vi "ExEMCircBufKinetics.vi"() -> ()   [LabVIEW 2010]
uses:
  CamHandle.vi
panel:
  out "Current clock index":u32
  out "current clock value":dbl format="%.2f"
  out "Min Clock index":u32
  out "Max Clock index":u32
  in  "Enum":T1(ring)
  in  "Vertical Clock":u32=2 min=1 max=16 step=1
  in  "Window Size":u32=50 min=1 step=1
  in  "av gain":dbl format="%.2f"
  in  "Invert Logic output":bool
  in  "Logic Output":i32
  in  "Fan":i32=1
  in  "ADC Gain":u32
  out "ADC Speed (Khz)":u32
  in  "Fast ADC":bool
  in  "Temperature":dbl=-70.0 format="%.2f"
  in  "Exposure":dbl min=0.0 step=0.001 format="%.3f"
  in  "stop":bool
  in  "Store":bool
  out "error out":errorcluster
  in  "error in (no error)":errorcluster
  # "ExEMCircBufKinetics:\nThis example allows a full image\nto be programmed up. It then runs\nin sync (focus) and kinetics mode displaying the full image made up\nof kinetic window exposures.\nNote: this example requires the \ncamera support circular buffers.\nThis example also shows how to \nsetup the cascade to run in over-\nlapped mode and how to set the\non-chip multiplication gain and how\nto set the readout port."
  # "Warning: you must open and run once the VI ExOpenGlobalCam.vi.\nYou only need to run it once then you can run this Example VI as many\ntimes as you want."
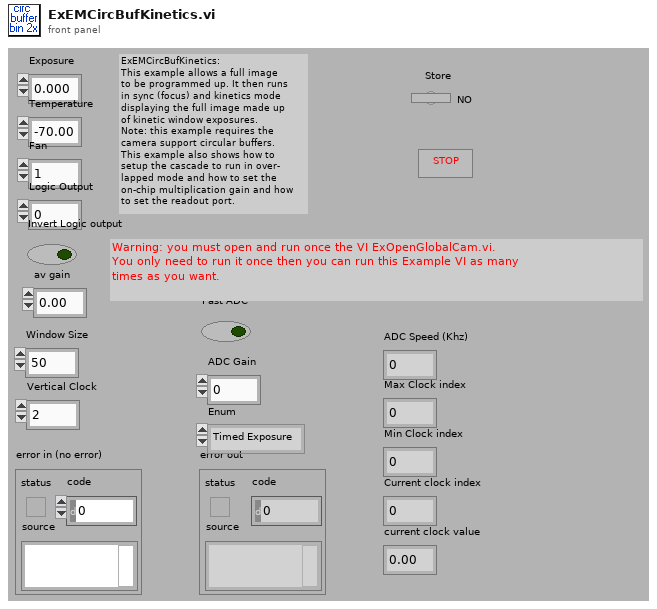
[diagram p1: front panel]
types:
  T1 = enum32{"Timed Exposure", "Trigger Once", "Trigger Multiple", "Trigger Bulb"}
  T2 = cluster{"Camera Handle":u32, "File Handle":u32, "Display Handle":u32, "Image Handle":u32}
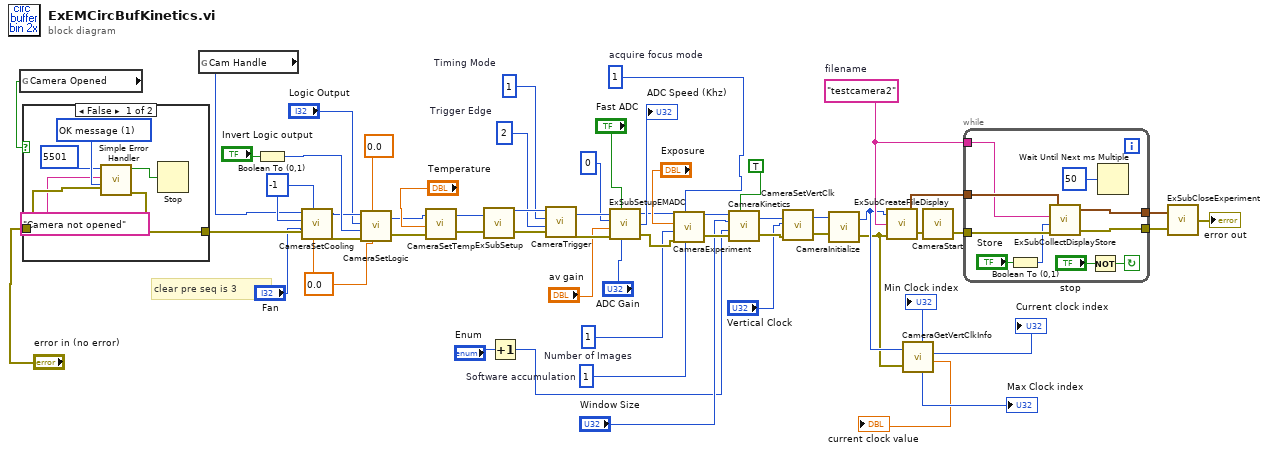
[diagram p0: block diagram]
diagram:
  w30 = 0.0
  w31 = -1
  w50 = u32 1  # Timing Mode
  w51 = u32 2  # Trigger Edge
  w19 = u32 1  # acquire focus mode
  w22 = u32 1  # Number of Images
  w18 = u32 1  # Software accumulation
  w59 = "testcamera2"  # filename
  # "clear pre seq is 3"
  n1 = global read "CamHandle.vi" "Camera Opened"() -> (w40:bool)
  n2 = case shown="False" w40 {
    tunnel: "error in (no error)" -> [w64 w66]
    tunnel: [w63 w66] -> w38
    frame False {
      w65 = u16 1 items=["no dialog", "OK message", "continue or stop message"] ("type of dialog (OK msg:1)")
      n3 = call <vilib>:"Simple Error Handler.vi"("error code (no error:0)"=5501, "error source (\" \")"="Camera not opened", "type of dialog (OK msg:1)"=w65, "error in (no error)"=w64) -> ("error?"=w61:bool, "error out"=w63:errorcluster)  [unwired: 1 in, 3 out]
      n4 = Stop(stop? (T)=w61) -> ()
    }
    frame True {
    }
  }
  n5 = global read "CamHandle.vi" "Cam Handle"() -> (w26:u32)
  n6 = Boolean To (0,1)(Boolean="Invert Logic output") -> (0, 1=w34:i16)
  n7 = call <userlib>:"CameraSetCooling.vi"("Reserved"=w30, "Cooling Mode"=w31, "error in (no error)"=w38, "Fan"="Fan", "Cooling"=w31, "Camera Handle"=w26) -> ("error out"=w37:errorcluster, "Camera Handle"=w33:u32)
  n8 = call <userlib>:"CameraSetLogic.vi"("Reserved 2"=w30, "Reserved"=0.0, "error in (no error)"=w37, "Invert Logic"=w34, "Logic Output"="Logic Output", "Camera Handle"=w33) -> ("error out"=w36:errorcluster, "Camera Handle"=w29:u32)
  n9 = call <userlib>:"CameraSetTemp.vi"("error in (no error)"=w36, "Temperature"="Temperature", "Camera Handle"=w29) -> ("error out"=w25:errorcluster, "Camera Handle"=w24:u32)
  n10 = call "ExSubSetup.vi"("error in (no error)"=w25, "Camera Handle"=w24) -> ("error out"=w48:errorcluster, "Camera Handle"=w54:u32)
  n11 = Increment(x="Enum") -> (x+1=w7:T1)
  n12 = call <userlib>:"CameraTrigger.vi"("error in"=w48, "Trigger Edge"=w51, "Timing Mode"=w50, "Camera Handle"=w54) -> ("error out"=w46:errorcluster, "Camera Handle"=w47:u32)
  n13 = call "ExSubSetupEMADC.vi"("Camera Handle"=w47, "Fast ADC"="Fast ADC", "ReadOut Port"=0, "Avalanche Gain\nOnly valid for \nport 0"="av gain", "ADC Gain"="ADC Gain", "error in (no error)"=w46) -> ("Camera Handle"=w20:u32, "ADC Speed (Khz)"=→"ADC Speed (Khz)":u32, "error out"=w23:errorcluster)
  n14 = call <userlib>:"CameraExperiment.vi"("Number of Accumulations"=w18, "Acquire / Focus Flag"=w19, "error in"=w23, "Number of Images"=w22, "Exposure (sec)"="Exposure", "Camera Handle"=w20) -> ("error out"=w17:errorcluster, "Camera Handle"=w16:u32)
  n15 = call <userlib>:"CameraKinetics.vi"("Camera Handle"=w16, "Window Size"="Window Size", "TriggerMode"=w7, "error in (no error)"=w17, "Enable/Disable Kinetics"=TRUE) -> ("Camera Handle"=w12:u32, "error out"=w13:errorcluster)
  n16 = call <userlib>:"CameraSetVertClk.vi"("error in (no error)"=w13, "Vertical Clock"="Vertical Clock", "Camera Handle"=w12) -> ("error out"=w10:errorcluster, "Camera Handle"=w9:u32)
  n17 = call <userlib>:"CameraInitialize.vi"("error in"=w10, "Camera Handle"=w9) -> ("error out"=w5:errorcluster, "Camera Handle"=w6:u32)
  n18 = call "ExSubCreateFileDisplay.vi"("error in (no error)"=w5, "File and Display Name"=w59, "Camera Handle"=w6) -> ("error out"=w52:errorcluster, "Handles Out"=w58:T2)
  n19 = call <userlib>:"CameraGetVertClkInfo.vi"("Camera Handle"=w6, "error in (no error)"=w5) -> ("Min"=→"Min Clock index":u32, "Max"=→"Max Clock index":u32, "VertClk index"=→"Current clock index":u32, "Real Clock Value"=→"current clock value":dbl)  [unwired: 2 out]
  n20 = call <userlib>:"CameraStart.vi"("error in"=w52) -> ("error out"=w53:errorcluster)  [unwired: 1 in, 1 out]
  n21 = while {
    tunnel: w58 -> [w75]
    tunnel: w53 -> [w74]
    tunnel: w59 -> [w67]
    tunnel: [w72] -> w56
    tunnel: [w73] -> w57
    stop <- w70 continue-if-true
    n22 = Boolean To (0,1)(Boolean="Store") -> (0, 1=w68:i16)
    n23 = call "ExSubCollectDisplayStore.vi"("error in (no error)"=w74, "Store flag"=w68, "Display Title"=w67, "Handle Cluster"=w75) -> ("error out"=w72:errorcluster, "Handle Cluster Out"=w73:T2)  [unwired: 1 out]
    n24 = Not(x="stop") -> (.not. x?=w70:bool)
    n25 = Wait Until Next ms Multiple(millisecond multiple=u32 50) -> ()  [unwired: 1 out]
  }
  n26 = call "ExSubCloseExperiment.vi"("error in (no error)"=w56, "Handles In"=w57) -> ("error out"=→"error out":errorcluster)
